vi "Create Pattern Script - Data Frame.vi"(8 "error in (no error)":errorcluster, 11 "BML Pattern Creater in":refnum<class "BML Pattern Creater.lvclass">) -> (0 "error out":errorcluster, 2 "Data Frame":string, 3 "BML Pattern Creater out":refnum<class "BML Pattern Creater.lvclass">)   [LabVIEW 2018, in "BML Pattern Creater.lvlib" / "BML Pattern Creater.lvclass"]
uses:
  BML Pattern Creater.lvclass
  BML Pattern Creater.lvclass/BML Pattern Creater.ctl
  Read Frame Data.vi
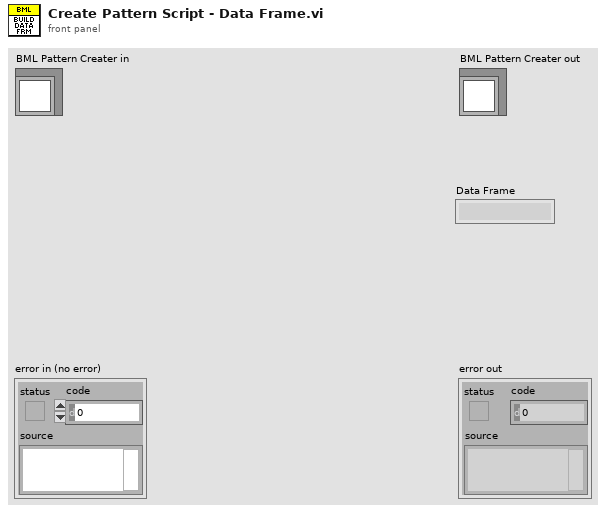
[diagram p1: front panel]
types:
  T1 = typedef "FRM Data - BML.ctl" = cluster{"Pattern_Name":string, "Data":u8[], "Start_Addr":u16, "ChipID":u8, "num of wait ms":i8, "Opcode":string[], "BML OM":T2, "BurstLength":T3, "FSN":u8, "R/W?":T4}
  T2 = typedef "OM - BML.ctl" = enum16{"Normal", "ImmeEffect", "InitSlaveID", "LoadData"}
  T3 = typedef "Burst Length.ctl" = enum8{"0", "2", "3", "4", "5", "8", "16", "32"}
  T4 = typedef "RW Options.ctl" = enum16{"Read", "Write", "R/W"}
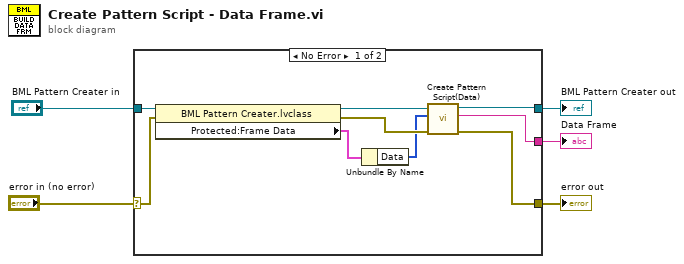
[diagram p0: block diagram]
diagram:
  n1 = case shown="No Error" "error in (no error)" {
    selector: "error in (no error)" -> [w13 w16]
    tunnel: [w7 w16] -> w4
    tunnel: [w8 w15] -> w2
    tunnel: "BML Pattern Creater in" -> [w14 w15]
    tunnel: [w6 _] -> w1
    frame No Error {
      n2 = property class="BML Pattern Creater.lvclass"(reference=w14, error in=w13) -> (reference out=w11:refnum<class "BML Pattern Creater.lvclass">, error out=w10:errorcluster, "Protected:Frame Data"=w12:T1)
      n3 = Unbundle By Name(w12) -> ("Data"=w9:u8[])
      n4 = call "Create Pattern Script(Data).vi"("error in (no error)"=w10, "Data"=w9, "BML Pattern Creater in"=w11) -> ("error out"=w7:errorcluster, "String"=w6:string, "BML Pattern Creater out"=w8:refnum<class "BML Pattern Creater.lvclass">)  [unwired: 6 in]
    }
    frame Error {
    }
  }
  "error out" <- w4
  "BML Pattern Creater out" <- w2
  "Data Frame" <- w1
